vi "Verify Environment.vi"(7 "소분류코드":string, 8 "error in (no error)":errorcluster caption="에러 입력(에러 없음)", 11 "교정환경":T1) -> (0 "error out":errorcluster caption="에러 출력", 2 "문자열":string, 3 "OK?":bool)   [LabVIEW 2020]
uses:
  Controls/Clst_Atm Info Global.ctl
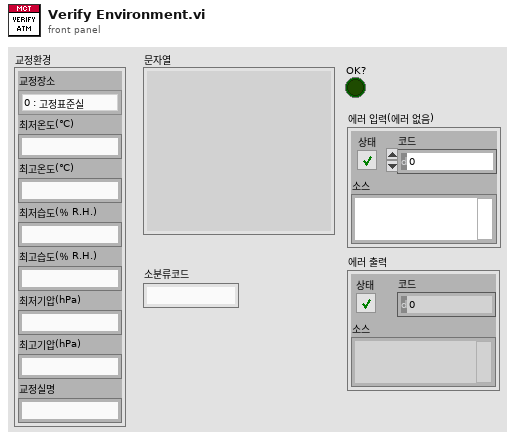
[diagram p1: front panel]
types:
  T1 = typedef "Clst_Atm Info Global.ctl" = cluster{"교정장소":enum16{"0 : 고정표준실", "1 : 현장교정"}, "최저온도(℃)":string, "최고온도(℃)":string, "최저습도(％ R.H.)":string, "최고습도(％ R.H.)":string, "최저기압(hPa)":string, "최고기압(hPa)":string, "교정실명":string}
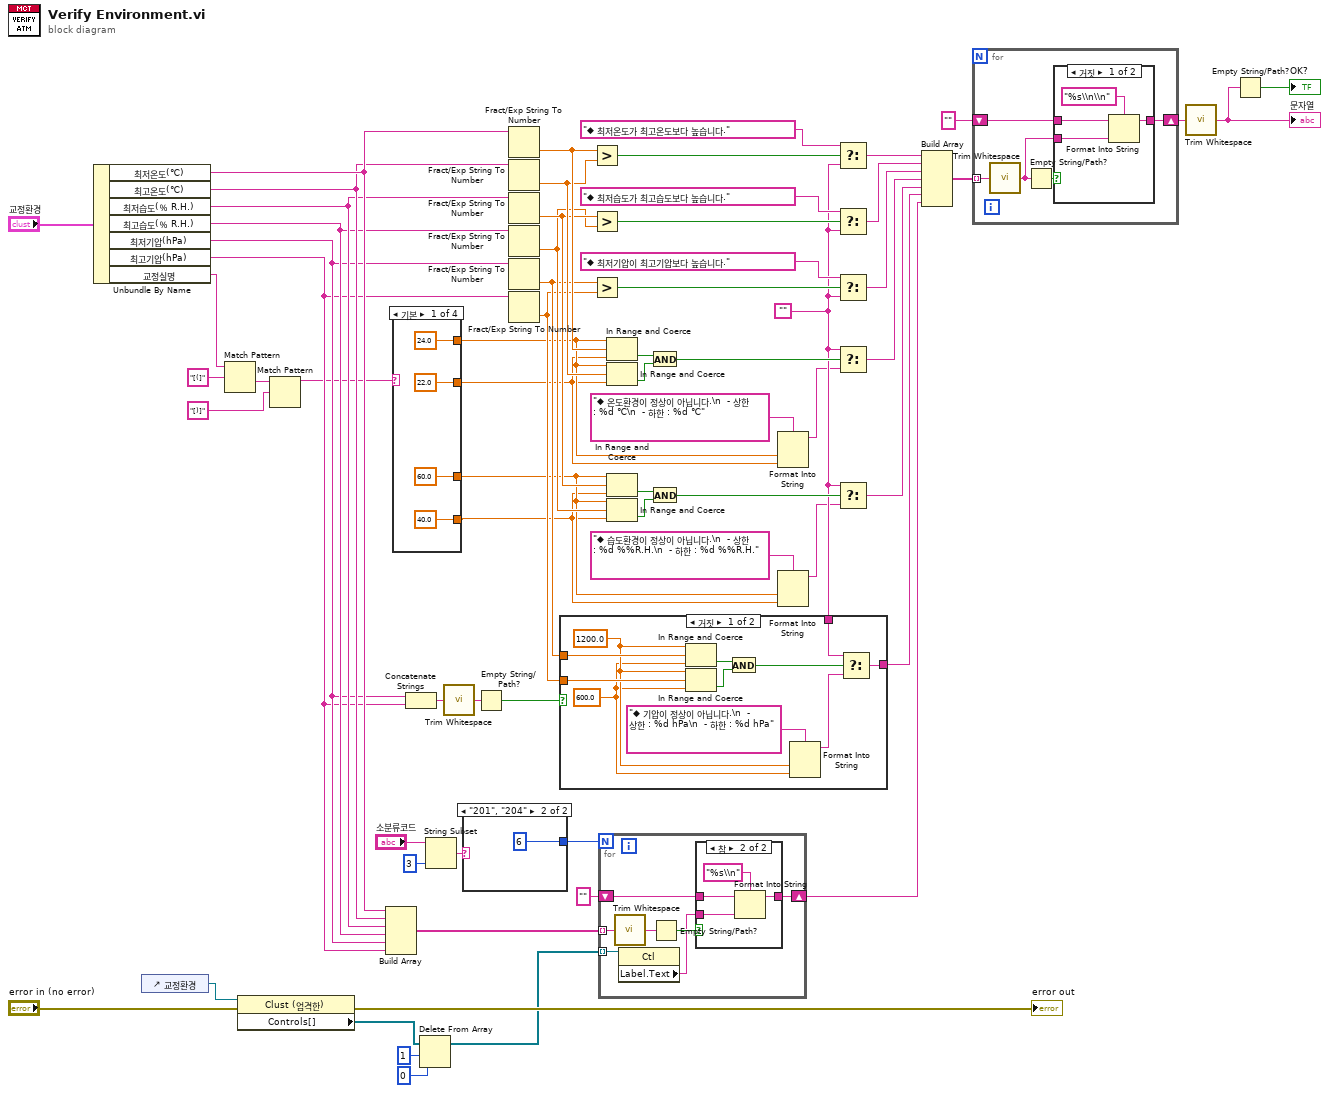
[diagram p0: block diagram]
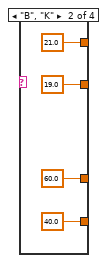
[diagram p2: hidden frame]
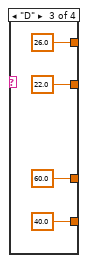
[diagram p3: hidden frame]
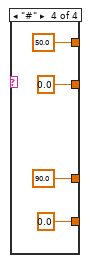
[diagram p4: hidden frame]
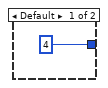
[diagram p5: hidden frame]
diagram:
  w47 = ""
  n1 = Unbundle By Name("교정환경") -> ("최저온도(℃)"=w34:string, "최고온도(℃)"=w33:string, "최저습도(％ R.H.)"=w32:string, "최고습도(％ R.H.)"=w31:string, "최저기압(hPa)"=w30:string, "최고기압(hPa)"=w29:string, "교정실명"=w14:string)
  n2 = control-ref of="교정환경"() -> (w27:refnum<vi>)
  n3 = Match Pattern(string=w14, regular expression="[(]" ("정규식")) -> (after substring=w12:string)  [unwired: 1 in, 3 out]
  n4 = property class="Clust (엄격한)"(reference=w27, error in="error in (no error)") -> (error out=→"error out":errorcluster, "Controls[]"=w18:refnum<vi>[])  [unwired: 1 out]
  n5 = Match Pattern(string=w12, regular expression="[)]" ("정규식")) -> (before substring=w10:string)  [unwired: 1 in, 3 out]
  n6 = Build Array(w34, w33, w32, w31, w30, w29) -> (w28:string[])
  n7 = case shown="기본" w10 {
    tunnel: [24.0 ("상위 리미트") 21.0 ("상위 리미트") 26.0 ("상위 리미트") 50.0 ("상위 리미트")] -> w7
    tunnel: [22.0 ("상위 리미트") 19.0 ("상위 리미트") 22.0 ("상위 리미트") 0.0 ("상위 리미트")] -> w6
    tunnel: [60.0 ("상위 리미트") 60.0 ("상위 리미트") 60.0 ("상위 리미트") 90.0 ("상위 리미트")] -> w3
    tunnel: [40.0 ("상위 리미트") 40.0 ("상위 리미트") 40.0 ("상위 리미트") 0.0 ("상위 리미트")] -> w2
    frame Default {
    }
    frame "B", "K" {
    }
    frame "D" {
    }
    frame "#" {
    }
  }
  n8 = Concatenate Strings(w30, w29) -> (w37:string)
  n9 = Delete From Array(array=w18, length=1 ("길이"), index=0 ("인덱스")) -> (array with subset deleted=w15:refnum<vi>[])  [unwired: 1 out]
  n10 = String Subset(string="소분류코드", length (rest)=3 ("길이(나머지)")) -> (substring=w21:string)  [unwired: 1 in]
  n11 = call <vilib>:"Trim Whitespace.vi"("string"=w37) -> ("trimmed string"=w36:string)  [unwired: 1 in]
  n12 = case shown="\"201\", \"204\"" w21 {
    tunnel: [4 6] -> w19
    frame Default {
    }
    frame "201", "204" {
    }
  }
  n13 = Empty String/Path?(string/path=w36) -> (empty?=w35:bool)
  n14 = Fract/Exp String To Number(string=w34) -> (number=w59:dbl)  [unwired: 3 in, 1 out]
  n15 = Fract/Exp String To Number(string=w33) -> (number=w58:dbl)  [unwired: 3 in, 1 out]
  n16 = Fract/Exp String To Number(string=w32) -> (number=w57:dbl)  [unwired: 3 in, 1 out]
  n17 = Fract/Exp String To Number(string=w31) -> (number=w56:dbl)  [unwired: 3 in, 1 out]
  n18 = Fract/Exp String To Number(string=w30) -> (number=w55:dbl)  [unwired: 3 in, 1 out]
  n19 = Fract/Exp String To Number(string=w29) -> (number=w54:dbl)  [unwired: 3 in, 1 out]
  n20 = case shown="거짓" w35 {
    tunnel: w55 -> [w96 _]
    tunnel: w54 -> [w95 _]
    tunnel: w47 -> [w91 w97]
    tunnel: [w90 w97] -> w41
    frame False {
      w86 = 600.0 ("상위 리미트")
      w87 = 1200.0 ("상위 리미트")
      n21 = In Range and Coerce(upper limit=w87, x=w96, lower limit=w86) -> (In Range?=w94:bool)  [unwired: 1 out]
      n22 = In Range and Coerce(upper limit=w87, x=w95, lower limit=w86) -> (In Range?=w93:bool)  [unwired: 1 out]
      n23 = And(x=w94, y=w93) -> (x .and. y?=w92:bool)
      n24 = Format Into String(format string="◆ 기압이 정상이 아닙니다.\n  - 상한 : %d hPa\n  - 하한 : %d hPa" ("메시지"), w87, w86) -> (resulting string=w88:string)  [unwired: 2 in, 1 out]
      n25 = Select(t=w91, s=w92, f=w88) -> (s? t:f=w90:string)
    }
    frame True {
    }
  }
  n26 = Greater?(x=w59, y=w58) -> (0:w66:bool)
  n27 = Greater?(x=w57, y=w56) -> (0:w63:bool)
  n28 = Greater?(x=w55, y=w54) -> (0:w61:bool)
  n29 = for {
    N: w19 -> [_]
    tunnel: w28 -> [w104] mode=indexing
    tunnel: w15 -> [w102] mode=indexing
    shift-right: [w99] -> w23
    shift-left: "" -> [w98]
    n30 = call <vilib>:"Trim Whitespace.vi"("string"=w104) -> ("trimmed string"=w103:string)  [unwired: 1 in]
    n31 = property class="Ctl"(reference=w102) -> ("Label.Text"=w100:string)  [unwired: 1 in, 2 out]
    n32 = Empty String/Path?(string/path=w103) -> (empty?=w101:bool)
    n33 = case shown="참" w101 {
      tunnel: w98 -> [w105 w108]
      tunnel: [w105 w109] -> w99
      tunnel: w100 -> [_ w106]
      frame False {
      }
      frame True {
        n34 = Format Into String(format string="%s\\n" ("포맷 문자열"), initial string=w108, w106) -> (resulting string=w109:string)  [unwired: 1 in, 1 out]
      }
    }
  }
  n35 = In Range and Coerce(upper limit=w7, x=w59, lower limit=w6) -> (In Range?=w53:bool)  [unwired: 1 out]
  n36 = In Range and Coerce(upper limit=w7, x=w58, lower limit=w6) -> (In Range?=w52:bool)  [unwired: 1 out]
  n37 = In Range and Coerce(upper limit=w3, x=w57, lower limit=w2) -> (In Range?=w50:bool)  [unwired: 1 out]
  n38 = In Range and Coerce(upper limit=w3, x=w56, lower limit=w2) -> (In Range?=w49:bool)  [unwired: 1 out]
  n39 = And(x=w53, y=w52) -> (x .and. y?=w51:bool)
  n40 = And(x=w50, y=w49) -> (x .and. y?=w48:bool)
  n41 = Format Into String(format string="◆ 온도환경이 정상이 아닙니다.\n  - 상한 : %d ℃\n  - 하한 : %d ℃" ("메시지"), w7, w6) -> (resulting string=w8:string)  [unwired: 2 in, 1 out]
  n42 = Format Into String(format string="◆ 습도환경이 정상이 아닙니다.\n  - 상한 : %d %%R.H.\n  - 하한 : %d %%R.H." ("메시지"), w3, w2) -> (resulting string=w4:string)  [unwired: 2 in, 1 out]
  n43 = Select(t="◆ 최저온도가 최고온도보다 높습니다." ("메시지"), s=w66, f=w47) -> (s? t:f=w46:string)
  n44 = Select(t="◆ 최저습도가 최고습도보다 높습니다." ("메시지"), s=w63, f=w47) -> (s? t:f=w45:string)
  n45 = Select(t="◆ 최저기압이 최고기압보다 높습니다." ("메시지"), s=w61, f=w47) -> (s? t:f=w44:string)
  n46 = Select(t=w47, s=w51, f=w8) -> (s? t:f=w43:string)
  n47 = Select(t=w47, s=w48, f=w4) -> (s? t:f=w42:string)
  n48 = Build Array(w46, w45, w44, w43, w42, w41, w23) -> (w40:string[])
  n49 = for {
    tunnel: w40 -> [w114] mode=indexing
    shift-right: [w111] -> w38
    shift-left: "" -> [w112]
    n50 = call <vilib>:"Trim Whitespace.vi"("string"=w114) -> ("trimmed string"=w110:string)  [unwired: 1 in]
    n51 = Empty String/Path?(string/path=w110) -> (empty?=w113:bool)
    n52 = case shown="거짓" w113 {
      tunnel: w112 -> [w117 w119]
      tunnel: [w118 w119] -> w111
      tunnel: w110 -> [w115 _]
      frame False {
        n53 = Format Into String(format string="%s\\n\\n" ("포맷 문자열"), initial string=w117, w115) -> (resulting string=w118:string)  [unwired: 1 in, 1 out]
      }
      frame True {
      }
    }
  }
  n54 = call <vilib>:"Trim Whitespace.vi"("string"=w38) -> ("trimmed string"=w1:string)  [unwired: 1 in]
  "문자열" <- w1
  n55 = Empty String/Path?(string/path=w1) -> (empty?=→"OK?":bool)
